vi "Read Loop.vi"(8 "error in (no error)":errorcluster, 9 "ReadElements":u32, 10 "Queues":T1, 11 "AODAcq in":refnum<class "AODAcq.lvclass">) -> (0 "error out":errorcluster, 3 "AODAcq out":refnum<class "AODAcq.lvclass">)   [LabVIEW 2012, in "AODAcq.lvclass"]
uses:
  AODAcq.lvclass
panel:
  out "Progress":dbl(slide) scale=0.0..1.0
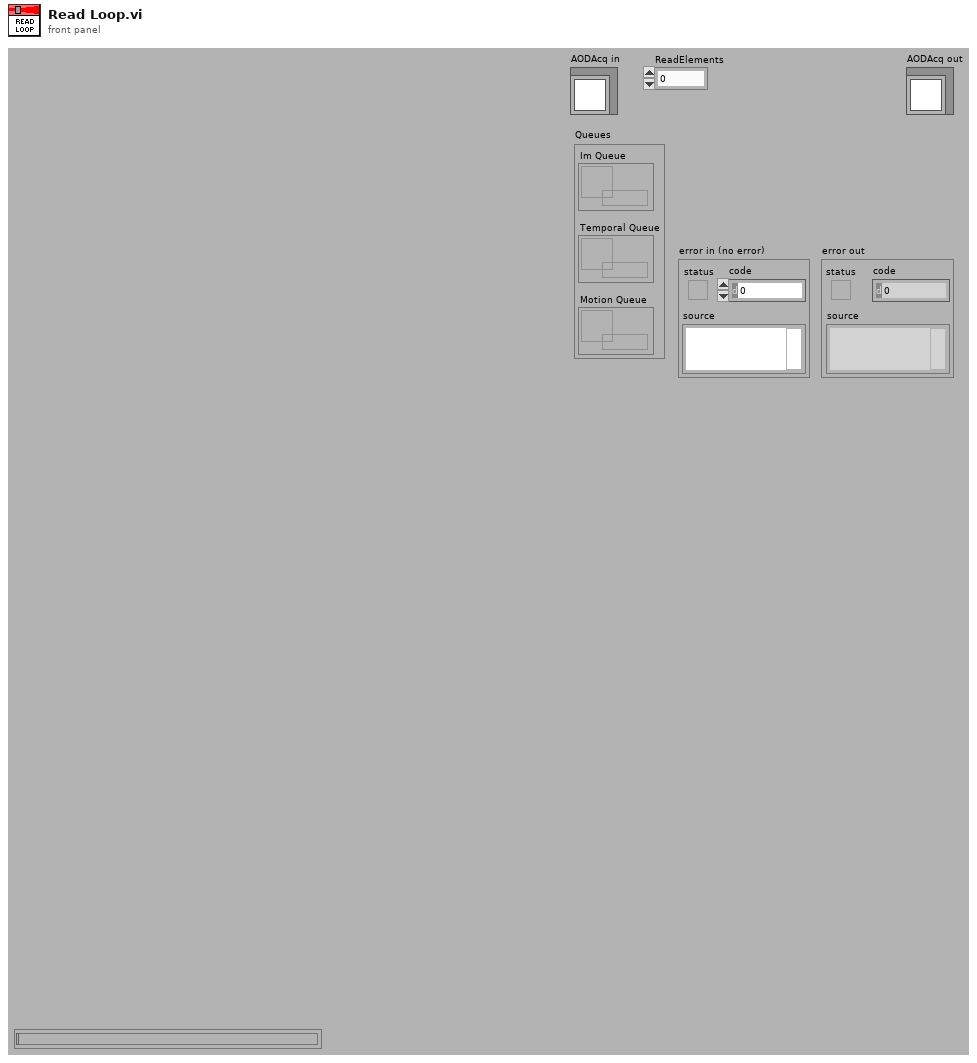
[diagram p1: front panel]
types:
  T1 = cluster{"Im Queue":refnum<queue>, "Temporal Queue":refnum<queue>, "Motion Queue":refnum<queue>}
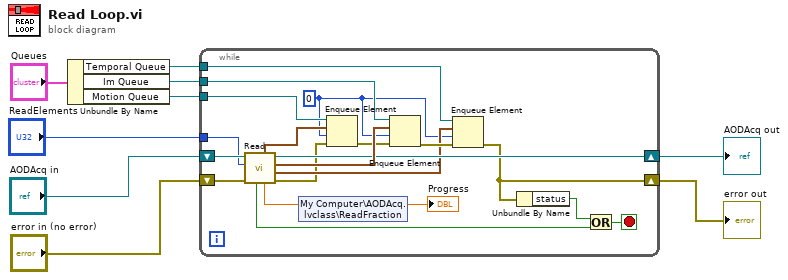
[diagram p0: block diagram]
diagram:
  n1 = Unbundle By Name("Queues") -> ("Temporal Queue"=w2:refnum<queue>, "Im Queue"=w1:refnum<queue>, "Motion Queue"=w3:refnum<queue>)
  n2 = while {
    tunnel: w1 -> [w26]
    tunnel: "ReadElements" -> [w23]
    shift-right: [w20] -> w6
    shift-left: "AODAcq in" -> [w28]
    shift-right: [w11] -> w8
    shift-left: "error in (no error)" -> [w27]
    tunnel: w2 -> [w16]
    tunnel: w3 -> [w14]
    stop <- w21 stop-if-true
    w10 = 0 ("timeout in ms (-1)")
    n3 = call-dynamic "Read.vi"("error in (no error)"=w27, "ReadElements"=w23, "AODAcq in"=w28) -> ("error out"=w13:errorcluster, "TemporalData"=w17:waveform(dbl)[], "ImData"=w25:waveform(i32)[], "AODAcq out"=w20:refnum<class "AODAcq.lvclass">, "ReadFraction"=w24:dbl, "MotionData"=w15:waveform(i32)[], "Done"=w19:bool)  [unwired: 2 in]
    "Progress" <- w24
    n4 = shared-variable "My Computer\\AODAcq.lvclass\\ReadFraction"(w24) -> ()  [unwired: 1 in, 1 out]
    n5 = Enqueue Element(queue=w14, element=w15, timeout in ms (-1)=w10, error in (no error)=w13) -> (error out=w12:errorcluster)  [unwired: 2 out]
    n6 = Enqueue Element(queue=w26, element=w25, timeout in ms (-1)=w10, error in (no error)=w12) -> (error out=w18:errorcluster)  [unwired: 2 out]
    n7 = Enqueue Element(queue=w16, element=w17, timeout in ms (-1)=w10, error in (no error)=w18) -> (error out=w11:errorcluster)  [unwired: 2 out]
    n8 = Unbundle By Name(w11) -> ("status"=w22:bool)
    n9 = Or(x=w22, y=w19) -> (x .or. y?=w21:bool)
  }
  "error out" <- w8
  "AODAcq out" <- w6
